vi "Get Property DataType.vi"(0 "SLSC Remote in":refnum<class "SLSC Remote.lvclass">, 5 "property":refnum<k21>, 11 "error in (no error)":errorcluster) -> (4 "SLSC Remote out":refnum<class "SLSC Remote.lvclass">, 6 "property out":refnum<k21>, 10 "Prop.DataType":i32(ring) items=["None", "Bool", "DBL", "I32", "I64", "String", "U32", "U64", "1D Bool", "1D DBL", "1D I32", "1D I64", "1D String", "1D U32", "1D U64"], 15 "error out":errorcluster)   [LabVIEW 2016, in "SLSC Interfaces.lvlib" / "SLSC Remote.lvclass"]
uses:
  SLSC Remote.lvclass
  C:/Users/tblair/Documents/Git Projects/SLSC-Interface/Source/SLSC Interface Class/SLSC Interface.lvclass
  <vilib>/National Instruments/JSON Support for LabVIEW/JSON Data Classes/JSON Object/JSON Object.lvclass
  C:/Program Files (x86)/National Instruments/LabVIEW 2016/vi.lib/National Instruments/JSON Support for LabVIEW/JSON Data Classes/JSON Datatype/JSON Datatype.lvclass
  <vilib>/National Instruments/JSON Support for LabVIEW/JSON Data Classes/JSON Object/New JSON Object (Empty).vi
  <vilib>/National Instruments/JSON Support for LabVIEW/JSON Data Classes/JSON Object/Insert Key Value Pair (Single String).vi
  <vilib>/NI/NI JSONRPC Server Framework/Classes/Server/Format Client Request (Auto-Increment).vi
  <vilib>/httpClient/POSTBuffer.vi
  <vilib>/National Instruments/JSON Support for LabVIEW/JSON Data Classes/JSON Datatype/To More Specific Type (Object).vi
  <vilib>/National Instruments/JSON Support for LabVIEW/JSON Data Classes/JSON Object/Get Value (String Value).vi
  <vilib>/NI/NI JSONRPC Server Framework/Classes/Server/JSONRPC Server.lvclass
  <vilib>/httpClient/LabVIEWHTTPClient.lvlib
  <vilib>/National Instruments/JSON Support for LabVIEW/JSON Data Classes/JSON Datatype/JSON Datatype.lvclass
  C:/Program Files (x86)/National Instruments/LabVIEW 2016/vi.lib/National Instruments/JSON Support for LabVIEW/JSON Data Classes/JSON Structured Type/JSON Structured Type.lvclass
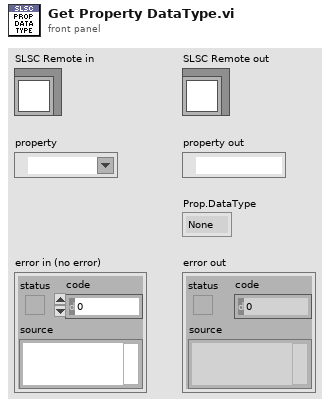
[diagram p1: front panel]
types:
  T1 = typedef "LabVIEWHTTPClient.lvlib/ClientHandle.ctl" = refnum<k1>
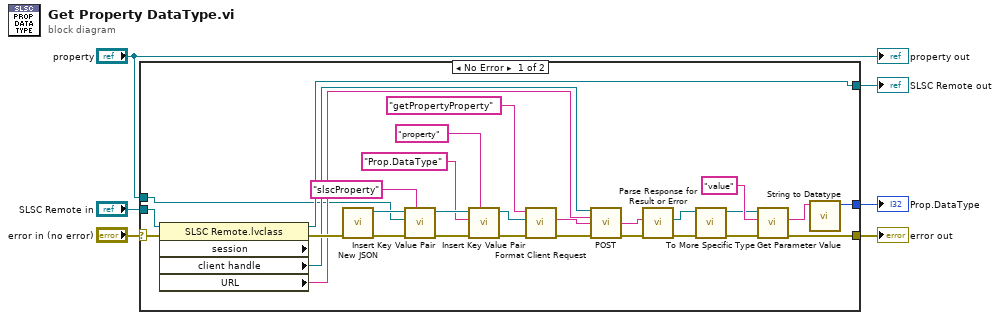
[diagram p0: block diagram]
diagram:
  n1 = case shown="No Error" "error in (no error)" {
    selector: "error in (no error)" -> [w33 w36]
    tunnel: "SLSC Remote in" -> [w35 w37]
    tunnel: [w34 w37] -> w2
    tunnel: [w22 w36] -> w4
    tunnel: "property" -> [w7 _]
    tunnel: [w17 _] -> w1
    frame No Error {
      n2 = property class="SLSC Remote.lvclass" props=["session", "client handle", "URL"](reference=w35, error in=w33) -> (reference out=w34:refnum<class "SLSC Remote.lvclass">, error out=w32:errorcluster, "client handle"=w28:T1, "URL"=w27:string)  [unwired: 1 out]
      n3 = call-poly <vilib>:"New JSON.vi"("error in (no error)"=w32) -> ("error out"=w31:errorcluster, "JSON Object out"=w12:refnum<class "JSON Object.lvclass">)  [unwired: 9 in]
      n4 = call-poly <vilib>:"Insert Key Value Pair.vi"("key"="slscProperty" ("Name"), "error in (no error)"=w31, "value"=w7, "JSON Object in"=w12) -> ("error out"=w18:errorcluster, "JSON Object out"=w11:refnum<class "JSON Object.lvclass">)  [unwired: 5 in, 1 out]
      n5 = call-poly <vilib>:"Insert Key Value Pair.vi"("key"="property" ("Name"), "error in (no error)"=w18, "value"="Prop.DataType" ("String"), "JSON Object in"=w11) -> ("error out"=w20:errorcluster, "JSON Object out"=w21:refnum<class "JSON Object.lvclass">)  [unwired: 5 in, 1 out]
      n6 = call-poly <vilib>:"Format Client Request.vi"("error in (no error)"=w20, "JSON in"=w21, "method"="getPropertyProperty") -> ("error out"=w26:errorcluster, "Request String"=w29:string)  [unwired: 7 in]
      n7 = call-poly <vilib>:"POST.vi"("client handle"=w28, "url"=w27, "buffer"=w29, "error in (no error)"=w26) -> ("body"=w25:string, "error out"=w24:errorcluster)  [unwired: 8 in, 2 out]
      n8 = call <vilib>:"Parse Response for Result or Error.vi"("error in"=w24, "Response String In"=w25) -> ("error out"=w23:errorcluster, "JSON out"=w14:refnum<class "JSON Datatype.lvclass">)  [unwired: 7 in, 1 out]
      n9 = call-poly <vilib>:"To More Specific Type.vi"("error in (no error)"=w23, "JSON Datatype in"=w14) -> ("error out"=w15:errorcluster, "JSON Datatype out"=w13:refnum<class "JSON Object.lvclass">)  [unwired: 8 in]
      n10 = call-poly <vilib>:"Get Parameter Value.vi"("error in (no error)"=w15, "key"="value" ("Parameter Name"), "JSON Object in"=w13) -> ("error out"=w22:errorcluster, "value"=w16:string)  [unwired: 6 in, 1 out]
      n11 = call "String to Datatype.vi"("String Value"=w16) -> ("Prop.DataType"=w17:i32)  [unwired: 10 in]
    }
    frame Error {
    }
  }
  "error out" <- w4
  "SLSC Remote out" <- w2
  "Prop.DataType" <- w1
  "property out" <- "property"
